vi "PrepareData4Graph.vi"(6 "Wavelength nm":dbl[](array[numeric])=[0.0, 1.0, 2.0, 3.0, 4.0, 5.0, 6.0], 7 "DataLF":T2(array[cluster]), 8 "AcqMode":T3(ring), 9 "Data type":T4(ring)) -> (1 "Spectrum":cluster{"Array 2":dbl[], "Array":dbl[]}(graph), 2 "Intensity Graph":dbl[][](graph), 4 "PLInt out":dbl[](array[numeric]), 5 "Wavelength out":dbl[](array[numeric]))   [LabVIEW 2019]
panel:
  out "Polarisation 1D Spectrum":cluster{"X":dbl, "Y":dbl}[](graph)
  in  "CCD ROI":T1(ring)
  out "ZDIM":i32
  in  "Image":dbl[][][](array[numeric])=[[[1.0, 2.0, 6.0, 4.0], [1.0, 3.0, 4.0, 2.0], [1.0, 4.0, 3.0, 1.0], [1.0, 5.0, 2.0, 5.0]]]
  out "XY Intensity Map":dbl[][](graph)
  in  "2D Data (PL vs FSM Pos)":dbl[][](array[numeric])
  in  "2D Data (PL vs Angle/WL)":dbl[][](array[numeric])
  in  "Angle":dbl[](array[numeric])
  out "Polarisation":dbl[][](graph)
  out "Wavelength_nm":dbl[](array[numeric])
  out "PLInt_cts":dbl[](array[numeric])
  out "YDIM":i32
  in  "2D Data (PL vs WL)":dbl[][](array[numeric])
  out "XDIM":i32
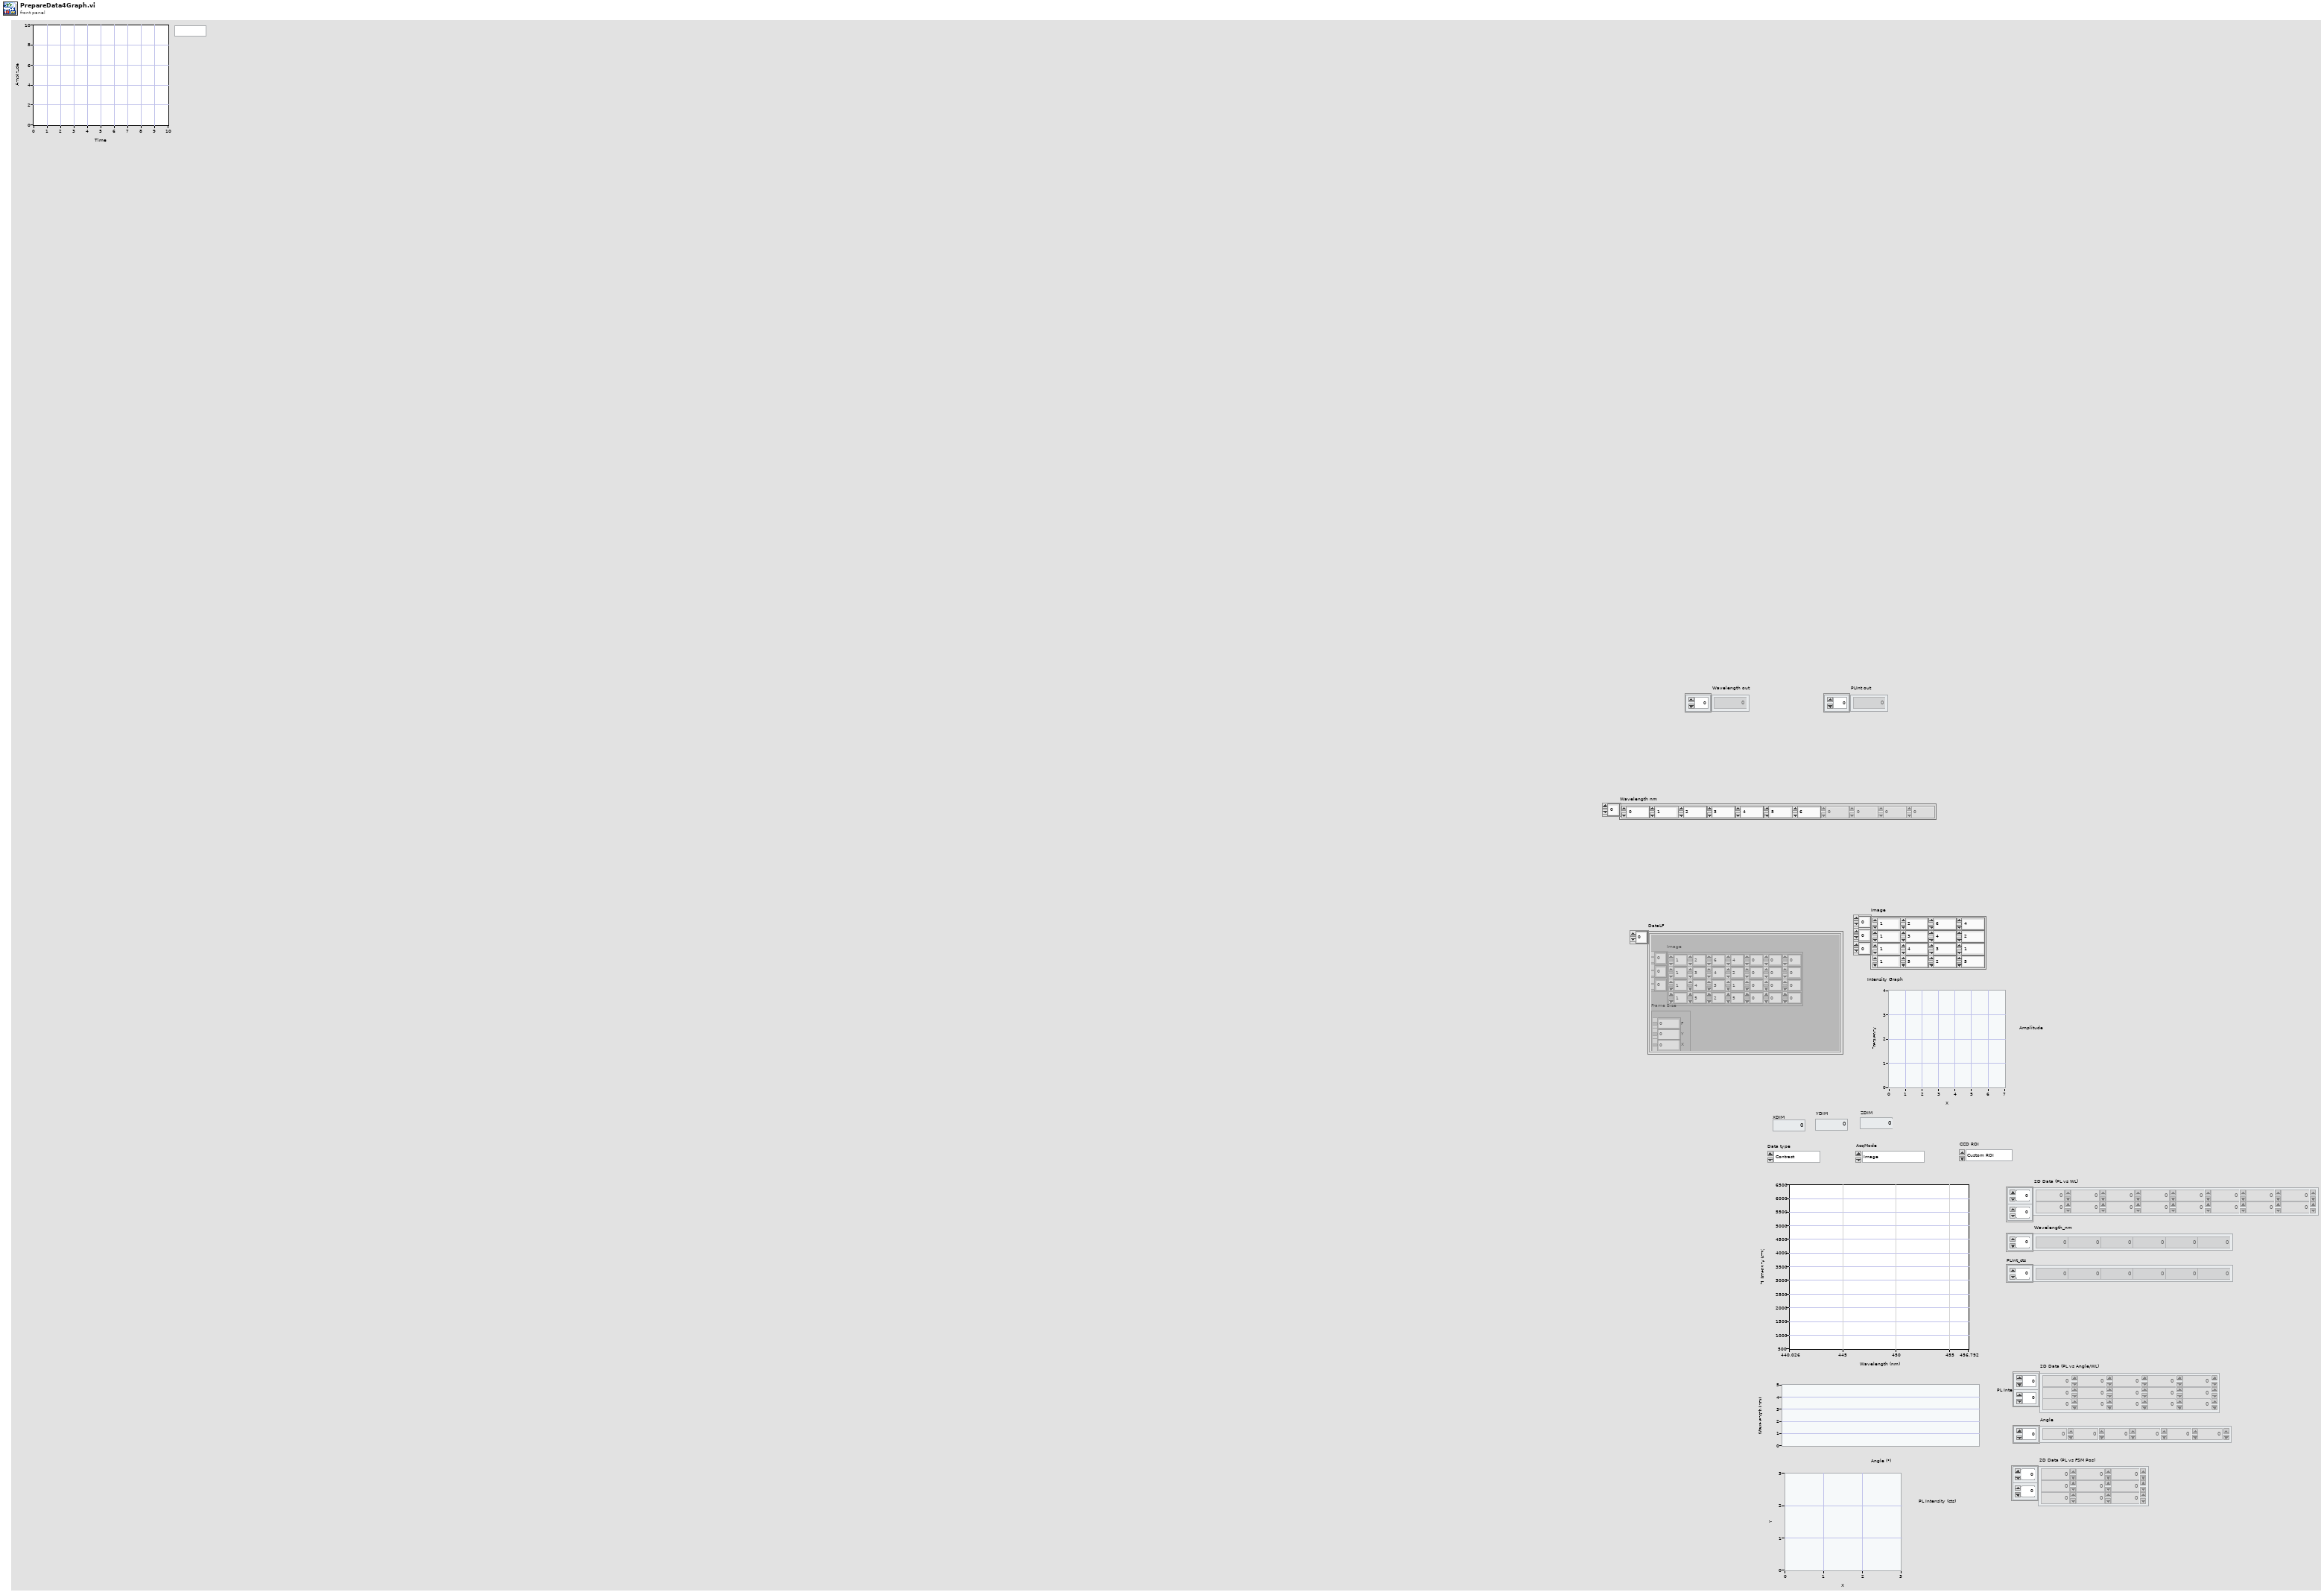
[diagram p1: front panel]
types:
  T1 = enum16{"Custom ROI", "Full sensor", "Binned full sensor"}
  T2 = cluster{"Image":dbl[][][], "Frame Size":cluster{"F":i32, "Y":i32, "X":i32}}[]
  T3 = enum16{"Image", "Spectrum", "APD 1", "APD 2", "APD 1+2"}
  T4 = enum16{"Contrast", "Spectre", "Polarisation", "XY Intensity Map"}
  T5 = cluster{"Image":dbl[][][], "Frame Size":cluster{"F":i32, "Y":i32, "X":i32}}
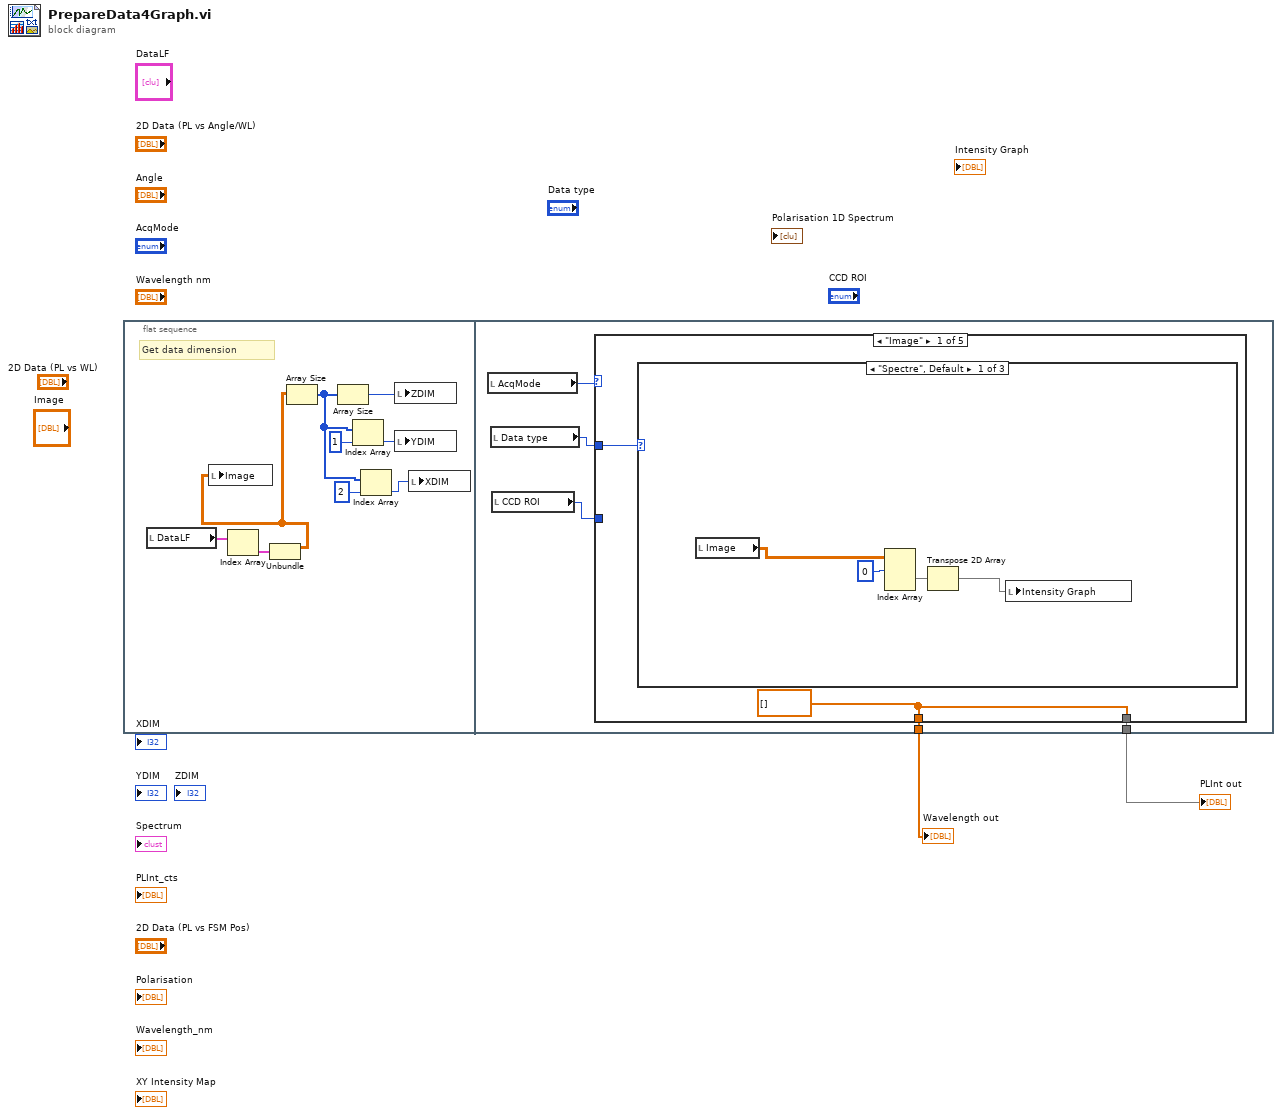
[diagram p0: block diagram]
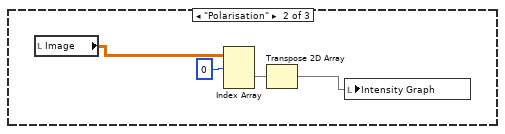
[diagram p2: hidden frame]
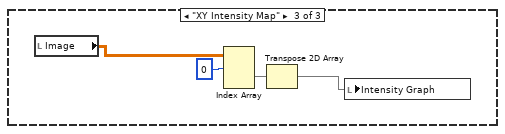
[diagram p3: hidden frame]
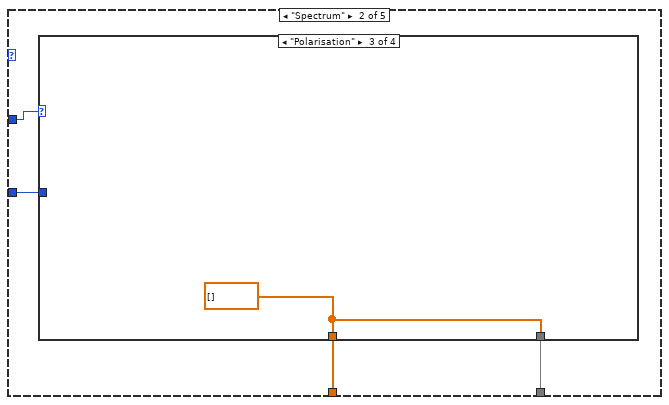
[diagram p4: hidden frame]
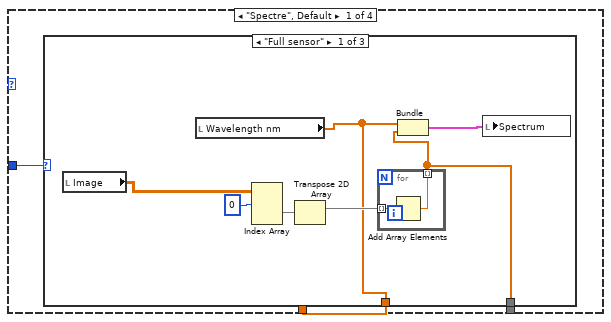
[diagram p5: hidden frame]
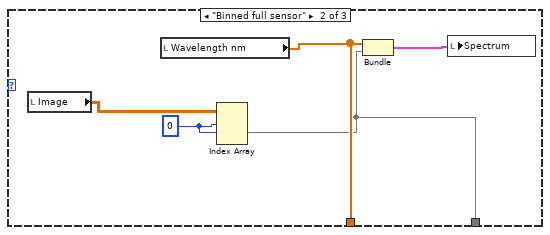
[diagram p6: hidden frame]
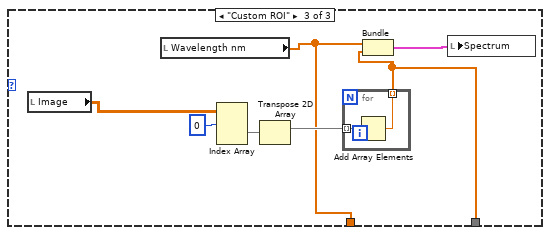
[diagram p7: hidden frame]
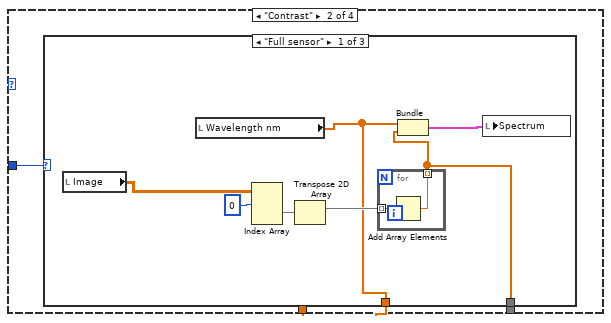
[diagram p8: hidden frame]
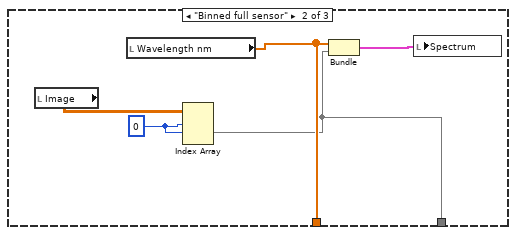
[diagram p9: hidden frame]
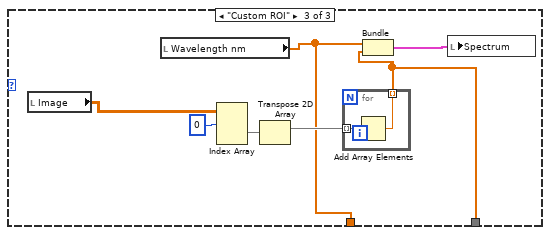
[diagram p10: hidden frame]
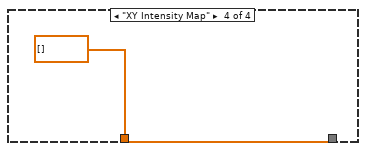
[diagram p11: hidden frame]
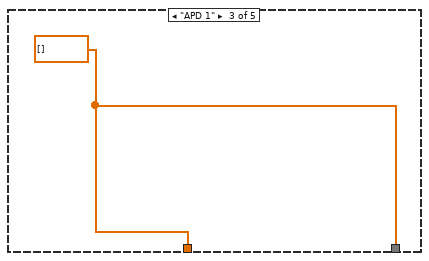
[diagram p12: hidden frame]
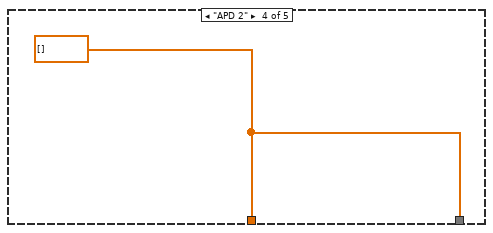
[diagram p13: hidden frame]
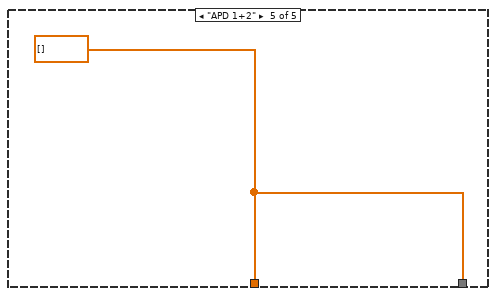
[diagram p14: hidden frame]
diagram:
  n1 = flat-sequence {
    tunnel: [w13] -> w2
    tunnel: [w12] -> w1
    frame #0 {
      # "Get data dimension"
      n2 = local read "DataLF"() -> (w5:T2)
      n3 = Index Array(array=w5) -> (element=w4:T5)  [unwired: 1 in]
      n4 = Unbundle(w4) -> ("Image"=w3:dbl[][][])  [unwired: 1 out]
      n5 = local write "Image"(w3) -> ()
      n6 = Array Size(array=w3) -> (size(s)=w7:i32[])
      n7 = Array Size(array=w7) -> (size(s)=w10:i32)
      n8 = Index Array(array=w7, index=1) -> (element=w9:i32)
      n9 = Index Array(array=w7, index=2) -> (element=w6:i32)
      n10 = local write "ZDIM"(w10) -> ()
      n11 = local write "YDIM"(w9) -> ()
      n12 = local write "XDIM"(w6) -> ()
    }
    frame #1 {
      n13 = local read "AcqMode"() -> (w16:T3)
      n14 = local read "Data type"() -> (w15:T4)
      n15 = local read "CCD ROI"() -> (w14:T1)
      n16 = case shown="\"Image\"" w16 {
        tunnel: w15 -> [w18 w34 _ _ _]
        tunnel: w14 -> [_ w33 _ _ _]
        tunnel: [w17 w32 w89 w90 w91] -> w13
        tunnel: [w17 w31 w89 w90 w91] -> w12
        frame "Image" {
          w17 = dbl[] []
          n17 = case shown="\"Spectre\", Default" w18 {
            frame "Spectre", Default {
              n18 = local read "Image"() -> (w20:dbl[][][])
              n19 = Index Array(array=w20, index (dim 0)=0 ("length")) -> (element=w22:dbl[][])  [unwired: 2 in]
              n20 = Transpose 2D Array(2D array=w22) -> (transposed array=w19:dbl[][])
              n21 = local write "Intensity Graph"(w19) -> ()
            }
            frame "Polarisation" {
              n22 = local read "Image"() -> (w24:dbl[][][])
              n23 = Index Array(array=w24, index (dim 0)=0 ("length")) -> (element=w26:dbl[][])  [unwired: 2 in]
              n24 = Transpose 2D Array(2D array=w26) -> (transposed array=w23:dbl[][])
              n25 = local write "Intensity Graph"(w23) -> ()
            }
            frame "XY Intensity Map" {
              n26 = local read "Image"() -> (w28:dbl[][][])
              n27 = Index Array(array=w28, index (dim 0)=0 ("length")) -> (element=w30:dbl[][])  [unwired: 2 in]
              n28 = Transpose 2D Array(2D array=w30) -> (transposed array=w27:dbl[][])
              n29 = local write "Intensity Graph"(w27) -> ()
            }
          }
        }
        frame "Spectrum" {
          n30 = case shown="\"Polarisation\"" w34 {
            tunnel: w33 -> [w37 w63 _ _]
            tunnel: [w36 w62 w87 w88] -> w32
            tunnel: [w35 w61 w87 w88] -> w31
            frame "Spectre", Default {
              n31 = case shown="\"Full sensor\"" w37 {
                tunnel: [w39 w48 w53] -> w36
                tunnel: [w38 w47 w52] -> w35
                frame "Full sensor" {
                  n32 = local read "Image"() -> (w40:dbl[][][])
                  n33 = local read "Wavelength nm"() -> (w39:dbl[])
                  n34 = Index Array(array=w40, index (dim 0)=0 ("length")) -> (element=w44:dbl[][])  [unwired: 2 in]
                  n35 = Transpose 2D Array(2D array=w44) -> (transposed array=w41:dbl[][])
                  n36 = for {
                    tunnel: w41 -> [w46] mode=indexing
                    tunnel: [w45] -> w38 mode=indexing
                    n37 = Add Array Elements(numeric array=w46) -> (sum=w45:dbl)
                  }
                  n38 = Bundle("Wavelength nm"=w39, w38) -> (w42:cluster{"Wavelength nm":dbl[], dbl[]})  [unwired: 1 in]
                  n39 = local write "Spectrum"(w42) -> ()
                }
                frame "Binned full sensor" {
                  w49 = 0 ("length")
                  n40 = local read "Image"() -> (w50:dbl[][][])
                  n41 = local read "Wavelength nm"() -> (w48:dbl[])
                  n42 = Index Array(array=w50, index (dim 0)=w49, index (dim 1)=w49) -> (element=w47:dbl[])  [unwired: 1 in]
                  n43 = Bundle("Wavelength nm"=w48, "Image"=w47) -> (w51:cluster{"Wavelength nm":dbl[], "Image":dbl[]})  [unwired: 1 in]
                  n44 = local write "Spectrum"(w51) -> ()
                }
                frame "Custom ROI" {
                  n45 = local read "Image"() -> (w54:dbl[][][])
                  n46 = local read "Wavelength nm"() -> (w53:dbl[])
                  n47 = Index Array(array=w54, index (dim 0)=0 ("length")) -> (element=w58:dbl[][])  [unwired: 2 in]
                  n48 = Transpose 2D Array(2D array=w58) -> (transposed array=w55:dbl[][])
                  n49 = for {
                    tunnel: w55 -> [w60] mode=indexing
                    tunnel: [w59] -> w52 mode=indexing
                    n50 = Add Array Elements(numeric array=w60) -> (sum=w59:dbl)
                  }
                  n51 = Bundle("Wavelength nm"=w53, w52) -> (w56:cluster{"Wavelength nm":dbl[], dbl[]})  [unwired: 1 in]
                  n52 = local write "Spectrum"(w56) -> ()
                }
              }
            }
            frame "Contrast" {
              n53 = case shown="\"Full sensor\"" w63 {
                tunnel: [w65 w74 w79] -> w62
                tunnel: [w64 w73 w78] -> w61
                frame "Full sensor" {
                  n54 = local read "Image"() -> (w66:dbl[][][])
                  n55 = local read "Wavelength nm"() -> (w65:dbl[])
                  n56 = Index Array(array=w66, index (dim 0)=0 ("length")) -> (element=w70:dbl[][])  [unwired: 2 in]
                  n57 = Transpose 2D Array(2D array=w70) -> (transposed array=w67:dbl[][])
                  n58 = for {
                    tunnel: w67 -> [w72] mode=indexing
                    tunnel: [w71] -> w64 mode=indexing
                    n59 = Add Array Elements(numeric array=w72) -> (sum=w71:dbl)
                  }
                  n60 = Bundle("Wavelength nm"=w65, w64) -> (w68:cluster{"Wavelength nm":dbl[], dbl[]})  [unwired: 1 in]
                  n61 = local write "Spectrum"(w68) -> ()
                }
                frame "Binned full sensor" {
                  w75 = 0 ("length")
                  n62 = local read "Image"() -> (w76:dbl[][][])
                  n63 = local read "Wavelength nm"() -> (w74:dbl[])
                  n64 = Index Array(array=w76, index (dim 0)=w75, index (dim 1)=w75) -> (element=w73:dbl[])  [unwired: 1 in]
                  n65 = Bundle("Wavelength nm"=w74, "Image"=w73) -> (w77:cluster{"Wavelength nm":dbl[], "Image":dbl[]})  [unwired: 1 in]
                  n66 = local write "Spectrum"(w77) -> ()
                }
                frame "Custom ROI" {
                  n67 = local read "Image"() -> (w80:dbl[][][])
                  n68 = local read "Wavelength nm"() -> (w79:dbl[])
                  n69 = Index Array(array=w80, index (dim 0)=0 ("length")) -> (element=w84:dbl[][])  [unwired: 2 in]
                  n70 = Transpose 2D Array(2D array=w84) -> (transposed array=w81:dbl[][])
                  n71 = for {
                    tunnel: w81 -> [w86] mode=indexing
                    tunnel: [w85] -> w78 mode=indexing
                    n72 = Add Array Elements(numeric array=w86) -> (sum=w85:dbl)
                  }
                  n73 = Bundle("Wavelength nm"=w79, w78) -> (w82:cluster{"Wavelength nm":dbl[], dbl[]})  [unwired: 1 in]
                  n74 = local write "Spectrum"(w82) -> ()
                }
              }
            }
            frame "Polarisation" {
              w87 = dbl[] []
            }
            frame "XY Intensity Map" {
              w88 = dbl[] []
            }
          }
        }
        frame "APD 1" {
          w89 = dbl[] []
        }
        frame "APD 2" {
          w90 = dbl[] []
        }
        frame "APD 1+2" {
          w91 = dbl[] []
        }
      }
    }
  }
  "Wavelength out" <- w2
  "PLInt out" <- w1
